vi "3.1.vi"(1 "数值":dbl) -> (0 "正弦":dbl, 2 "余弦":dbl)   [LabVIEW 2017]
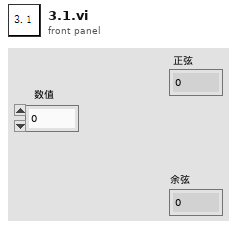
[diagram p1: front panel]
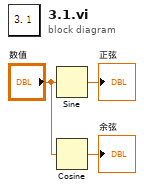
[diagram p0: block diagram]
diagram:
  n1 = Sine(x="数值") -> (sin(x)=→"正弦":dbl)
  n2 = Cosine(x="数值") -> (cos(x)=→"余弦":dbl)
